vi "GetDataType.vi"(8 "error in":errorcluster, 11 "Tunnel in":refnum<class "Tunnel.lvclass">) -> (0 "error out":errorcluster, 2 "Data Type":variant, 3 "Tunnel out":refnum<class "Tunnel.lvclass">)   [LabVIEW 2014, in "Raspberry Pi Compatible Compiler for LabVIEW.lvlib" / "Tunnel.lvclass"]
uses:
  Tunnel.lvclass
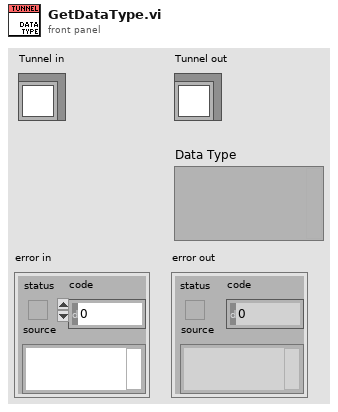
[diagram p1: front panel]
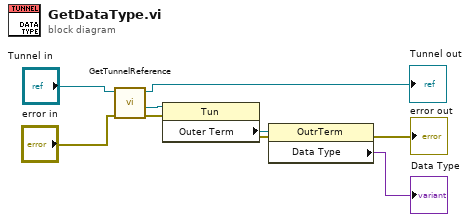
[diagram p0: block diagram]
diagram:
  n1 = call "GetTunnelReference.vi"("error in"="error in", "Tunnel in"="Tunnel in") -> ("error out"=w8:errorcluster, "reference out"=w9:refnum<vi>, "Tunnel out"=→"Tunnel out":refnum<class "Tunnel.lvclass">)  [unwired: 7 in]
  n2 = property class="Tun"(reference=w9, error in=w8) -> (error out=w6:errorcluster, "Outer Term"=w5:refnum<vi>)  [unwired: 1 out]
  n3 = property class="OutrTerm"(reference=w5, error in=w6) -> (error out=→"error out":errorcluster, "Data Type"=→"Data Type":variant)  [unwired: 1 out]
